vi "Intake Constants.vi"() -> ()   [LabVIEW 2018]
panel:
  in  "Peak Reverse":dbl=0.3
  in  "Peak Forward":dbl=0.2
  in  "Turn Travel\nUnits Per Rotation":dbl=3600.0
  in  "Rotations\nTo Travel":dbl=6.0
  in  "Gain 4":T1={"kP"=0.0, "kI "=0.0, "kD"=0.0, "kF"=0.0, "I Zone"=0.0, "Peak Out"=1.0}
  in  "Gain 3":T1={"kP"=0.0, "kI "=0.0, "kD"=0.0, "kF"=0.0, "I Zone"=0.0, "Peak Out"=1.0}
  in  "Gain 2":T1={"kP"=0.0, "kI "=0.0, "kD"=0.0, "kF"=0.0, "I Zone"=0.0, "Peak Out"=1.0}
  in  "PID Gains":T1={"kP"=5.5, "kI "=0.021, "kD"=0.0, "kF"=0.2436, "I Zone"=50.0, "Peak Out"=1.0}
  in  "Neutral\nDeadband":dbl=0.001
  in  "Timeout Ms":i32=10
  in  "Encoder Units\nPer Rotation":i32=15884
  in  "Sensor Units\nPer Rotation":i32=1440
  in  "Gain 4 Slot":i32=3
  in  "Gain 3 Slot":i32=2
  in  "Gain 2 Slot":i32=1
  in  "PID Slot":i32
  in  "PID Turn":i32=1
  in  "PID Primary":i32
  # "How many\nsensor units\nper rotation:\nCTRE Mag\nEncoder"
  # "Empirically\nmeasure the\ndifference\nbetween \nencoders per\n360 degrees"
  # "Scales units to\n3600 per rotation.\nThis is nice, as it\nmeans one unit is\n0.1 degrees."
  # "Constants"
  # "You shouldn't need\nto change these"
  # "0 - Skip confirmation\nNonZero - Wait and log\nto DS if something fails"
  # "Motor's\nNeutral deadband"
  # "0.1504411764705882 = 1023/6800"
  # "1023 = Max Output\n6800 = Measured Max Output"
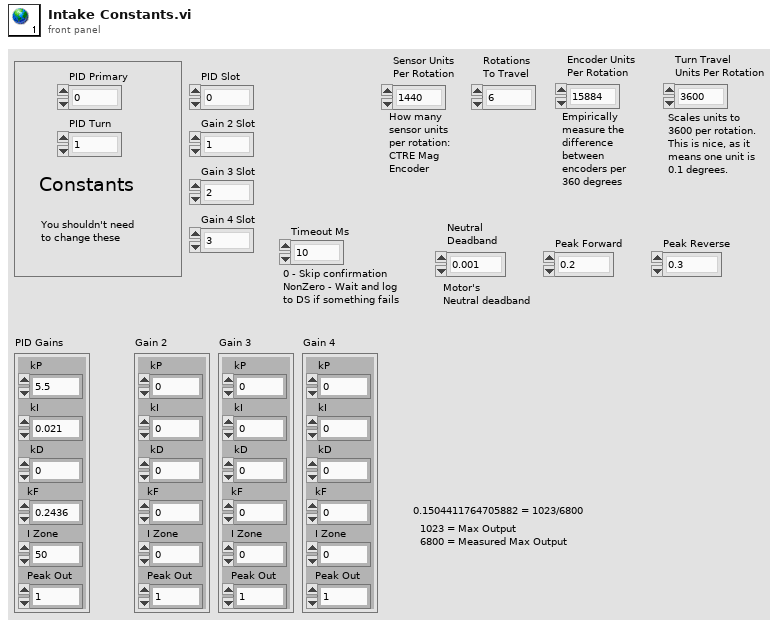
[diagram p1: front panel]
types:
  T1 = cluster{"kP":dbl, "kI ":dbl, "kD":dbl, "kF":dbl, "I Zone":dbl, "Peak Out":dbl}
diagram:
